vi "Read Amplitude.vi"(8 "error in (no error)":errorcluster, 11 "Lock-in worker in":refnum<class "Lock-in worker.lvclass">) -> (0 "error out":errorcluster, 2 "Amplitude":dbl, 3 "Lock-in worker out":refnum<class "Lock-in worker.lvclass">)   [LabVIEW 2015, in "Lock-in worker.lvclass"]
uses:
  Lock-in worker.lvclass
  Lock-in worker.lvclass/Lock-in worker.ctl
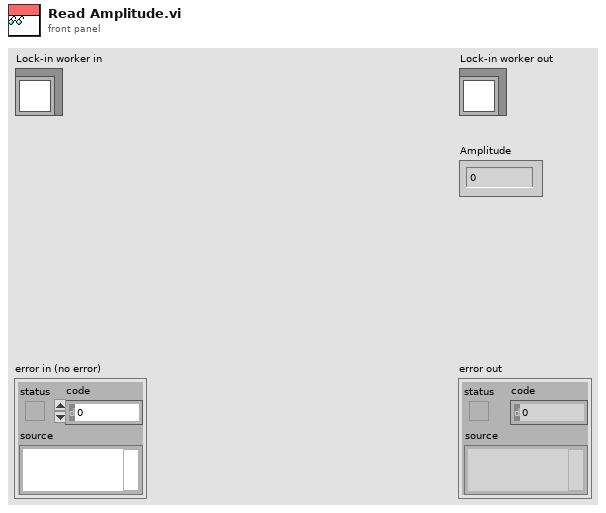
[diagram p1: front panel]
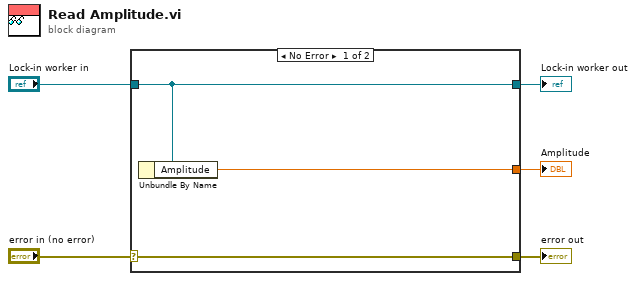
[diagram p0: block diagram]
diagram:
  n1 = case shown="No Error" "error in (no error)" {
    selector: "error in (no error)" -> [w8 w9]
    tunnel: [w8 w9] -> w4
    tunnel: [w7 w10] -> w2
    tunnel: "Lock-in worker in" -> [w7 w10]
    tunnel: [w6 _] -> w1
    frame No Error {
      n2 = Unbundle By Name(w7) -> ("Amplitude"=w6:dbl)
    }
    frame Error {
    }
  }
  "error out" <- w4
  "Lock-in worker out" <- w2
  "Amplitude" <- w1
